vi "Test DAQ.vi"() -> ()   [LabVIEW 2024]
panel:
  in  "Delay Time (s)":dbl=1.0
  in  "Numeric":i32=1
  out "data out":cluster{dbl, dbl, dbl, dbl}={-0.04345703125, 1.3466796875, -0.000244140625, 0.000244140625}
  out "relative seconds":dbl=20.251949199999217 format="%_19f"
  in  "Step":dbl=0.2 format="%#_13g"
  out "error out":errorcluster
  in  "Init Voltage":dbl=1.0
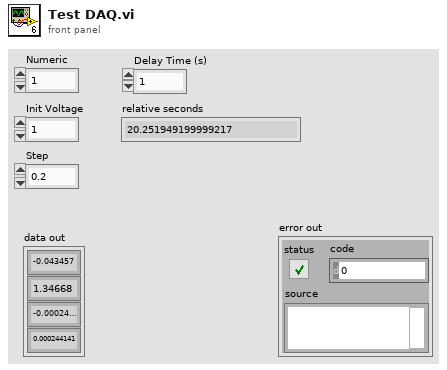
[diagram p1: front panel]
types:
  T1 = cluster{"AI0":dbl, "AI1":dbl, "AI2":dbl, "AI3":dbl}
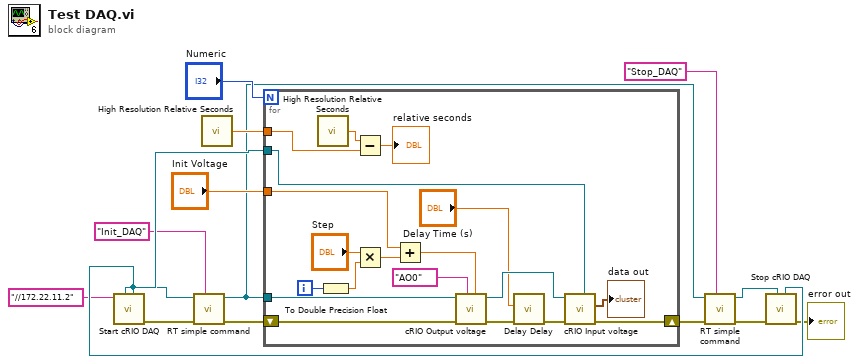
[diagram p0: block diagram]
diagram:
  n1 = call "Start cRIO DAQ.vi"("cRIO IP"="//172.22.11.2") -> ("error out"=w10:errorcluster, "DAQ_AI_Reader endpoint"=w14:refnum<k21>, "DAQ_CMD_Writer endpoint"=w9:refnum<k21>)  [unwired: 8 in]
  n2 = call "RT simple command.vi"("Command"="Init_DAQ", "error in (no error)"=w10, "DAQ_CMD_Writer endpoint"=w9) -> ("error out"=w7:errorcluster, "DAQ_CMD_Writer endpoint out"=w5:refnum<k21>)  [unwired: 7 in]
  n3 = call <vilib>:"High Resolution Relative Seconds.vi"() -> ("relative seconds"=w11:dbl)
  n4 = for {
    N: "Numeric" -> [_]
    tunnel: w5 -> [w34]
    tunnel: "Init Voltage" -> [w25]
    tunnel: w14 -> [w29]
    shift-right: [w16] -> w6
    shift-left: w7 -> [w32]
    tunnel: w11 -> [w20]
    i -> [w28]
    n5 = call <vilib>:"High Resolution Relative Seconds.vi"() -> ("relative seconds"=w21:dbl)
    n6 = To Double Precision Float(number=w28) -> (double precision float=w26:dbl)
    n7 = Subtract(x=w21, y=w20) -> (x-y=→"relative seconds":dbl)
    n8 = Multiply(x="Step", y=w26) -> (x*y=w24:dbl)
    n9 = Add(x=w25, y=w24) -> (x+y=w23:dbl)
    n10 = call "cRIO Output voltage.vi"("Voltage"=w23, "AO Channel"="AO0", "error in (no error)"=w32, "DAQ_CMD_Writer endpoint"=w34) -> ("error out"=w19:errorcluster, "DAQ_CMD_Writer endpoint out"=w30:refnum<k21>)  [unwired: 6 in]
    n11 = call "Delay Delay"("error in (no error)"=w19, "Delay Time (s)"="Delay Time (s)") -> ("error out"=w17:errorcluster)  [unwired: 9 in]
    n12 = call "cRIO Input voltage.vi"("DAQ_AI_Reader endpoint"=w29, "error in (no error)"=w17, "DAQ_CMD_Writer endpoint"=w30) -> ("error out"=w16:errorcluster, "output cluster"=→"data out":T1)  [unwired: 6 in, 1 out]
  }
  n13 = call "RT simple command.vi"("Command"="Stop_DAQ", "error in (no error)"=w6, "DAQ_CMD_Writer endpoint"=w5) -> ("error out"=w3:errorcluster, "DAQ_CMD_Writer endpoint out"=w4:refnum<k21>)  [unwired: 7 in]
  n14 = call "Stop cRIO DAQ.vi"("DAQ_AI_Reader endpoint"=w14, "DAQ_CMD_Writer endpoint"=w4, "error in (no error)"=w3) -> ("error out"=→"error out":errorcluster)  [unwired: 8 in]
